vi "UTIL Clear Session Data.vi"(0 "niDTS Test in":refnum<class "niDTS Comm Serial.lvclass">, 11 "error in":errorcluster) -> (4 "niDTS Test out":refnum<class "niDTS Comm Serial.lvclass">, 15 "error out":errorcluster)   [LabVIEW 2015, in "niDTS CommLib.lvlib" / "niDTS Comm Serial.lvclass"]
doc: "OVERRIDE VI\nPlaceholder for decendant classes to clear session information and close references."
uses:
  niDTS Comm Serial.lvclass
  String_class/niDTS Comm String.lvclass
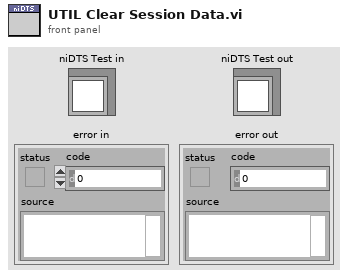
[diagram p1: front panel]
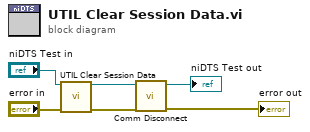
[diagram p0: block diagram]
diagram:
  n1 = call-parent "UTIL Clear Session Data.vi"("niDTS Test in"="niDTS Test in", "error in"="error in") -> ("niDTS Test out"=w4:refnum<class "niDTS Comm Serial.lvclass">, "error out"=w3:errorcluster)  [unwired: 12 in]
  n2 = call-dynamic "Comm Disconnect.vi"("error in (no error)"=w3, "niDTS Comm Serial in"=w4) -> ("error out"=→"error out":errorcluster, "niDTS Comm Serial out"=→"niDTS Test out":refnum<class "niDTS Comm Serial.lvclass">)  [unwired: 8 in]
